vi "Configure Digital Gen MLS.vi"(5 "Enable Waveform (T: Enable)":bool=TRUE, 6 "Enable Pinking Filter (T: Enable)":bool=TRUE, 7 "Sequence Length (15)":i32=15, 8 "error in (no error)":errorcluster, 9 "Amplitude (0 FFS)":dbl, 10 "Channel (0: chA)":i32(ring) items=["chA", "chB"], 11 "VISA resource name":refnum<visa-resource-name>) -> (0 "error out":errorcluster, 3 "VISA resource name out":refnum<visa-resource-name>)   [LabVIEW 2014, in "Stanford Research SR1.lvlib"]
doc: "Configures the attributes for the Digital Generator MLS."
uses:
  Stanford Research SR1.lvlib
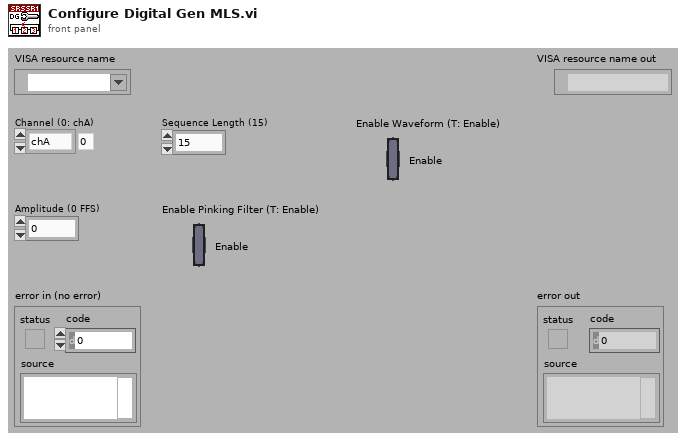
[diagram p1: front panel]
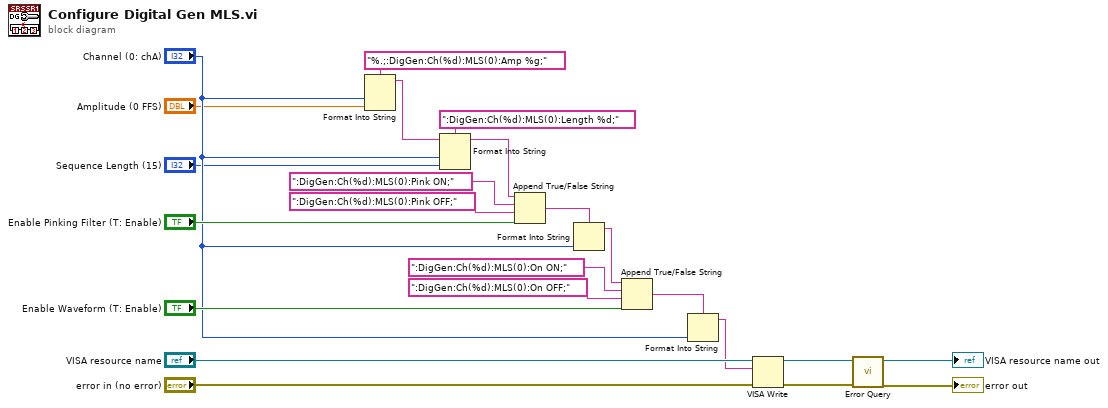
[diagram p0: block diagram]
diagram:
  n1 = Format Into String(format string="%.;:DigGen:Ch(%d):MLS(0):Amp %g;", "Channel (0: chA)", "Amplitude (0 FFS)") -> (resulting string=w22:string)  [unwired: 2 in, 1 out]
  n2 = Format Into String(format string=":DigGen:Ch(%d):MLS(0):Length %d;", initial string=w22, "Channel (0: chA)", "Sequence Length (15)") -> (resulting string=w20:string)  [unwired: 1 in, 1 out]
  n3 = Append True/False String(1:"Enable Pinking Filter (T: Enable)", 2:":DigGen:Ch(%d):MLS(0):Pink OFF;", 3:":DigGen:Ch(%d):MLS(0):Pink ON;", 4:w20) -> (0:w7:string)
  n4 = Format Into String(format string=w7, "Channel (0: chA)") -> (resulting string=w6:string)  [unwired: 2 in, 1 out]
  n5 = Append True/False String(1:"Enable Waveform (T: Enable)", 2:":DigGen:Ch(%d):MLS(0):On OFF;", 3:":DigGen:Ch(%d):MLS(0):On ON;", 4:w6) -> (0:w5:string)
  n6 = Format Into String(format string=w5, "Channel (0: chA)") -> (resulting string=w4:string)  [unwired: 2 in, 1 out]
  n7 = VISA Write(VISA resource name="VISA resource name", write buffer=w4, error in (no error)="error in (no error)") -> (VISA resource name out=w11:refnum<visa-resource-name>, error out=w10:errorcluster)  [unwired: 1 out]
  n8 = call "Error Query.vi"("error in (no error)"=w10, "VISA resource name"=w11) -> ("error out"=→"error out":errorcluster, "VISA resource name out"=→"VISA resource name out":refnum<visa-resource-name>)  [unwired: 6 in, 2 out]
